vi "SaveImage_local.vi"(1 "File Path":path, 2 "Color Palette":cluster{"Red":u8, "Green":u8, "Blue":u8}[](array[cluster]), 3 "Image":T1) -> ()   [LabVIEW 2013]
uses:
  <vilib>/vision/Image Controls.llb/IMAQ Image.ctl
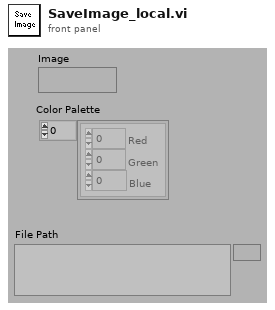
[diagram p1: front panel]
types:
  T1 = typedef "IMAQ Image.ctl" = refnum<image>
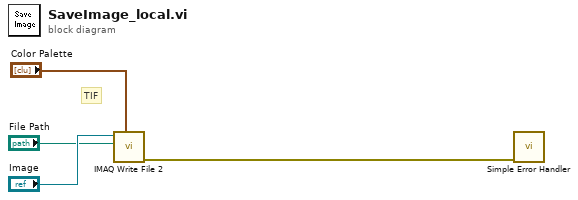
[diagram p0: block diagram]
diagram:
  # "TIF"
  n1 = call-poly "IMAQ Write File 2"("Color Palette"="Color Palette", "File Path"="File Path", "Image"="Image") -> ("error out"=w1:errorcluster)  [unwired: 2 in, 6 out]
  n2 = call <vilib>:"Simple Error Handler.vi"("error in (no error)"=w1) -> ()  [unwired: 1 in, 8 out]
